vi "例6.2 利用二进制文件IO进行数据保存保存与读取.vi"() -> ()   [LabVIEW 2017]
panel:
  out "读取的数据":T1
  in  "要保存的数据":T1={"班级名称"="203班", "学生成绩"=[], "平均分"=95.0, "是否通过"=FALSE}
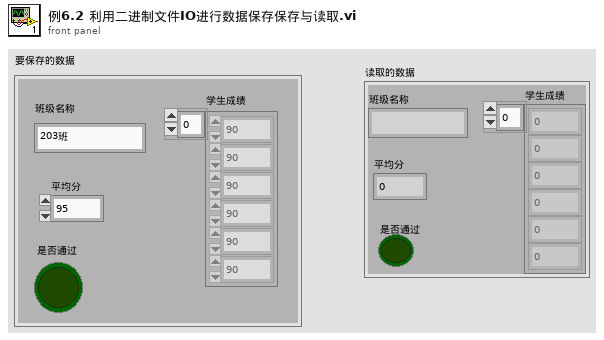
[diagram p1: front panel]
types:
  T1 = cluster{"班级名称":string, "学生成绩":dbl[], "平均分":dbl, "是否通过":bool}
  T2 = enum16{"open", "replace", "create", "open or create", "replace or create", "replace or create with confirmation"}
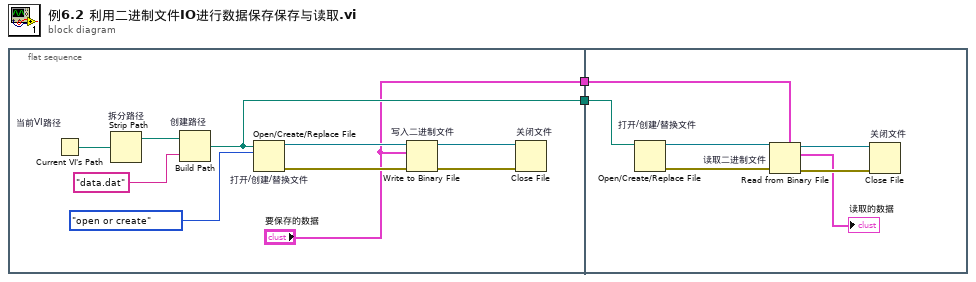
[diagram p0: block diagram]
diagram:
  n1 = flat-sequence {
    tunnel: ["要保存的数据"] -> w2
    tunnel: [w6] -> w1
    tunnel: w2 -> [w19]
    tunnel: w1 -> [w18]
    frame #0 {
      n2 = Current VI's Path "当前VI路径"() -> (path=w12:path)
      n3 = Strip Path "拆分路径"(path=w12) -> (stripped path=w11:path)  [unwired: 1 out]
      n4 = Build Path "创建路径"(base path=w11, name or relative path="data.dat" ("名称或相对路径")) -> (appended path=w6:path)
      n5 = Open/Create/Replace File "打开/创建/替换文件"(file path (use dialog)=w6, operation (0:open)=T2."open or create" ("操作(0:open)")) -> (refnum out=w7:refnum<file>, error out=w8:errorcluster)  [unwired: 4 in, 1 out]
      n6 = Write to Binary File "写入二进制文件"(file (use dialog)=w7, data="要保存的数据", error in=w8) -> (refnum out=w5:refnum<file>, error out=w4:errorcluster)  [unwired: 3 in, 1 out]
      n7 = Close File "关闭文件"(refnum=w5, error in=w4) -> ()  [unwired: 2 out]
    }
    frame #1 {
      n8 = Open/Create/Replace File "打开/创建/替换文件"(file path (use dialog)=w18) -> (refnum out=w17:refnum<file>, error out=w16:errorcluster)  [unwired: 5 in, 1 out]
      n9 = Read from Binary File "读取二进制文件"(5:w19, 8:w16, 11:w17) -> (0:w14:errorcluster, 2:→"读取的数据":T1, 3:w15:refnum<file>)  [unwired: 3 in, 1 out]
      n10 = Close File "关闭文件"(refnum=w15, error in=w14) -> ()  [unwired: 2 out]
    }
  }
